vi "groups_and_names_query.vi"(8 "error in (no error)":errorcluster, 10 "Small?":bool, 11 "Constraints":T1 {"Estimate Quality" scale=0.0..5.0}) -> (0 "error out":errorcluster, 1 "Description":string, 2 "Groups":string[](array[string]), 3 "Names":string[](array[string]), 4 "Description Returned?":bool)   [LabVIEW 2015]
doc: "Returns all groups and experiments within the given constraints and (if there is only one group) returns a description of the group and all experiments within the constraints."
uses:
  User Interface/Controls/Constraints.ctl
  <userlib>/_OpenG.lib/array/array.llb/Remove Duplicates from 1D Array (String)__ogtk.vi
  <userlib>/_OpenG.lib/array/array.llb/Empty 2D Array (Variant)__ogtk.vi
  <vilib>/addons/database/_DB Variant To Data/Database Variant To Data.xnode
panel:
  out "Min-Max experiment settings query":string
  out "Names SQL Query":string
  out "Selected Group":string
  out "Groups SQL Query":string
  out "Description SQL Query":string
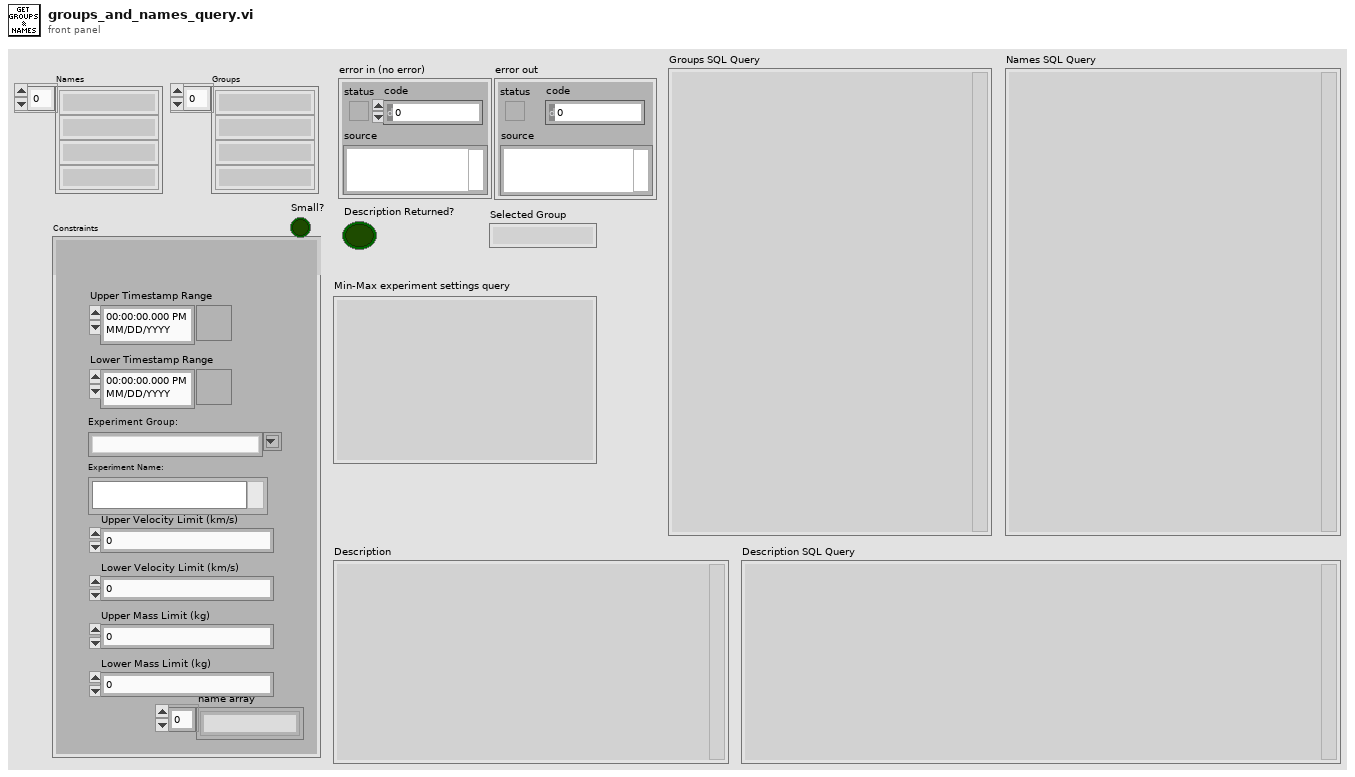
[diagram p1: front panel]
types:
  T1 = typedef "Constraints.ctl" = cluster{"Upper Timestamp Range":timestamp, "Lower Timestamp Range":timestamp, "Experiment Group:":string, "Experiment Name:":i32[], "Upper Velocity Limit (km/s)":dbl, "Lower Velocity Limit (km/s)":dbl, "Upper Mass Limit (kg)":dbl, "Lower Mass Limit (kg)":dbl, "name array":string[], "Estimate Quality":cluster{dbl, dbl}}
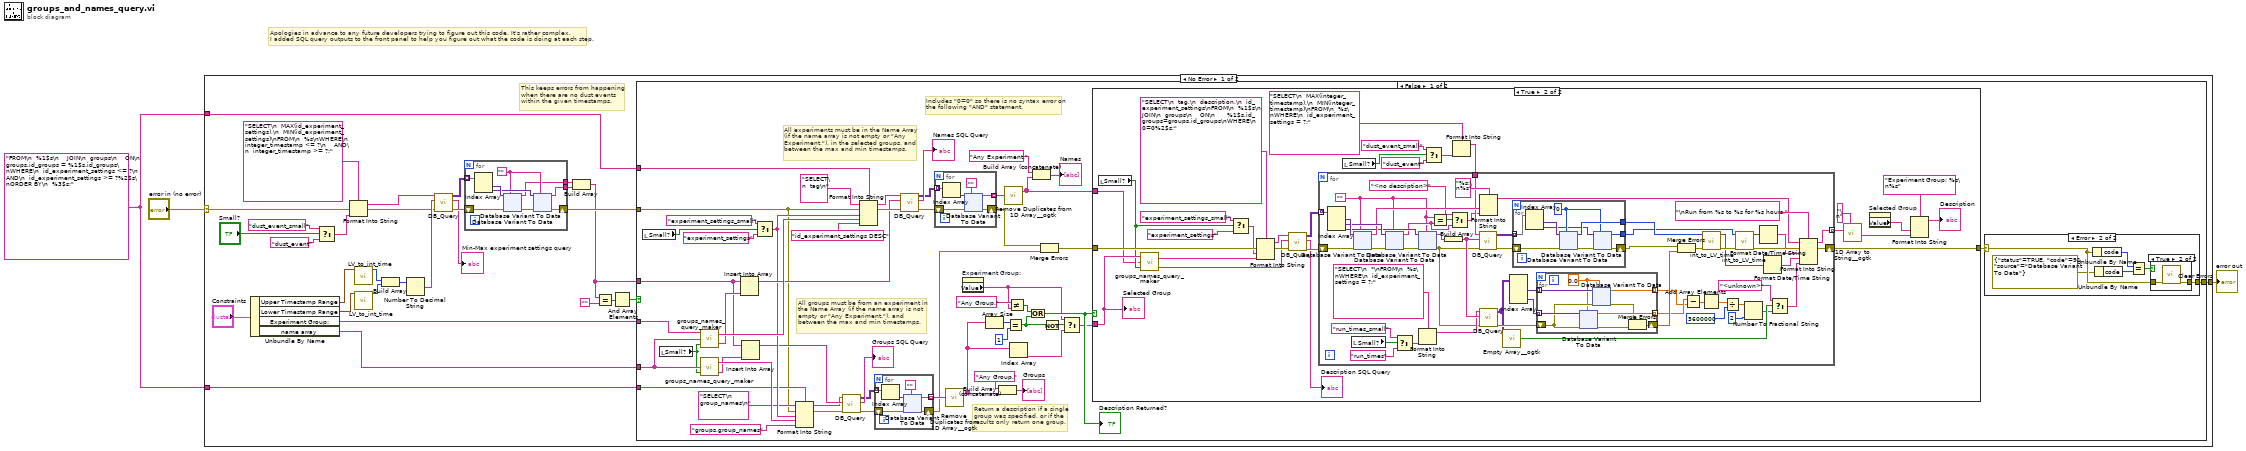
[diagram p0: block diagram]
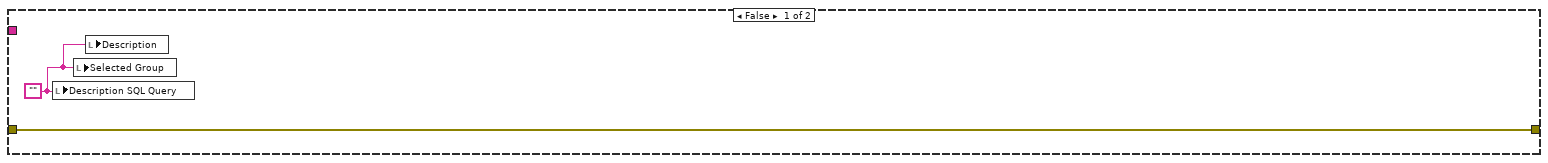
[diagram p4: hidden frame]
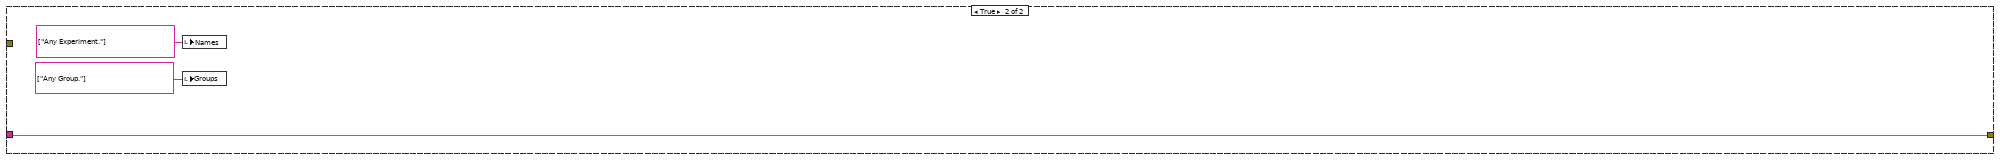
[diagram p5: hidden frame]
diagram:
  w1 = "FROM\n  %1$s\n    JOIN\n  groups\n    ON\n      groups.id_groups = %1$s.id_groups\nWHERE\n  id_experiment_settings <= ?\n    AND\n  id_experiment_settings >= ?%2$s\nORDER BY\n  %3$s;" ("format string")
  # "Apologies in advance to any future developers trying to figure out this code. It's rather complex.\nI added SQL query outputs to the front panel to help you figure out what the code is doing at each step."
  n1 = case shown="No Error" "error in (no error)" {
    selector: "error in (no error)" -> [w17 w578]
    tunnel: [w33 w578] -> w3
    tunnel: w1 -> [w22 _]
    tunnel: w1 -> [w21 _]
    frame No Error {
      # "This keeps errors from happening\nwhen there are no dust events\nwithin the given timestamps."
      n2 = Unbundle By Name("Constraints") -> ("Upper Timestamp Range"=w31:timestamp, "Lower Timestamp Range"=w32:timestamp, "Experiment Group:"=w20:string, "name array"=w29:string[])
      n3 = Select(t="dust_event_small", s="Small?", f="dust_event") -> (s? t:f=w18:string)
      n4 = Format Into String(format string="SELECT\n  MAX(id_experiment_settings),\n  MIN(id_experiment_settings)\nFROM\n  %s\nWHERE\n  integer_timestamp <= ?\n    AND\n  integer_timestamp >= ?;", error in=w17, w18) -> (resulting string=w15:string, error out=w14:errorcluster)  [unwired: 1 in]
      n5 = call "LV_to_int_time.vi"("Time Stamp"=w31) -> ("Integer Time"=w26:i64)  [unwired: 8 in, 1 out]
      n6 = call "LV_to_int_time.vi"("Time Stamp"=w32) -> ("Integer Time"=w25:i64)  [unwired: 8 in, 1 out]
      n7 = Build Array(w26, w25) -> (w24:i64[])
      n8 = Number To Decimal String(number=w24) -> (decimal integer string=w16:string[])  [unwired: 1 in]
      n9 = call "DB_Query.vi"("error in (no error)"=w14, "Parameters"=w16, "Parameterized Query"=w15) -> ("error out"=w13:errorcluster, "Query in Standard Format"=→"Min-Max experiment settings query":string, "Results"=w12:variant[][])  [unwired: 6 in]
      n10 = for {
        shift-right: [w507] -> w11
        shift-left: w13 -> [w512]
        tunnel: w12 -> [w513] mode=indexing
        tunnel: [w506] -> w10
        tunnel: [w505] -> w9
        w508 = "" ("t")
        n11 = Index Array(array=w513) -> (element #1=w511:variant, element #2=w509:variant)  [unwired: 2 in]
        n12 = xnode "Database Variant To Data"("database variant"=w511, "error in (no error)"=w512, "type"=w508) -> ("data"=w506:string, "error out"=w510:errorcluster)
        n13 = xnode "Database Variant To Data"("database variant"=w509, "error in (no error)"=w510, "type"=w508) -> ("data"=w505:string, "error out"=w507:errorcluster)
      }
      n14 = Build Array(w10, w9) -> (w7:string[])
      n15 = Equal?(x=w7, y="") -> (x = y?=w4:bool[])
      n16 = And Array Elements(Boolean array=w4) -> (logical AND=w5:bool)
      n17 = case shown="False" w5 {
        tunnel: [w87 w504] -> w33
        tunnel: w29 -> [w67 _]
        tunnel: w22 -> [w42 _]
        tunnel: w21 -> [w41 _]
        tunnel: w20 -> [w40 _]
        tunnel: w11 -> [w36 w504]
        tunnel: w7 -> [w35 _]
        frame False {
          # "Includes \"0=0\" so there is no syntax error on\nthe following \"AND\" statement."
          # "Return a description if a single\ngroup was specified, or if the\nresults only return one group."
          # "All groups must be from an experiment in\nthe Name Array (if the name array is not\nempty or \"Any Experiment.\"), and\nbetween the max and min timestamps."
          # "All experiments must be in the Name Array\n(if the name array is not empty or \"Any\nExperiment.\"), in the selected groups, and\nbetween the max and min timestamps."
          n18 = local read "Small?"() -> (w37:bool)
          n19 = local read "Small?"() -> (w38:bool)
          n20 = call "groups_names_query_maker.vi"("Small?"=w38, "Name Array"=w67) -> ("Parameters"=w54:string[], "Group and Names Query"=w55:string)  [unwired: 1 in]
          n21 = call "groups_names_query_maker.vi"("Small?"=w38, "Name Array"=w67, "Group  Name"=w40) -> ("Parameters"=w61:string[], "Group and Names Query"=w64:string)
          n22 = Insert Into Array(array=w35, new element=w61) -> (w58:string[])  [unwired: 1 in]
          n23 = Insert Into Array(array=w35, new element=w54) -> (w52:string[])  [unwired: 1 in]
          n24 = Select(t="experiment_settings_small", s=w37, f="experiment_settings") -> (s? t:f=w56:string)
          n25 = Format Into String(format string=w41, initial string="SELECT\n  group_names\n", error in=w36, w56, w55, "groups.group_names" ("input 4")) -> (resulting string=w51:string, error out=w53:errorcluster)
          n26 = call "DB_Query.vi"("error in (no error)"=w53, "Parameters"=w52, "Parameterized Query"=w51) -> ("error out"=w48:errorcluster, "Query in Standard Format"=→"Groups SQL Query":string, "Results"=w49:variant[][])  [unwired: 6 in]
          n27 = Format Into String(format string=w42, initial string="SELECT\n  tag\n", error in=w36, w56, w64, "id_experiment_settings DESC" ("input 4")) -> (resulting string=w63:string, error out=w62:errorcluster)
          n28 = for {
            tunnel: [w466] -> w84 mode=indexing
            shift-right: [w465] -> w81
            shift-left: w48 -> [w469]
            tunnel: w49 -> [w464] mode=indexing
            n29 = Index Array(array=w464) -> (element=w467:variant)  [unwired: 1 in]
            n30 = xnode "Database Variant To Data"("database variant"=w467, "error in (no error)"=w469, "type"="" ("t")) -> ("data"=w466:string, "error out"=w465:errorcluster)
          }
          n31 = call "DB_Query.vi"("error in (no error)"=w62, "Parameters"=w58, "Parameterized Query"=w63) -> ("error out"=w57:errorcluster, "Query in Standard Format"=→"Names SQL Query":string, "Results"=w59:variant[][])  [unwired: 6 in]
          n32 = for {
            tunnel: [w89] -> w85 mode=indexing
            shift-right: [w90] -> w82
            shift-left: w57 -> [w93]
            tunnel: w59 -> [w88] mode=indexing
            n33 = Index Array(array=w88) -> (element=w91:variant)  [unwired: 1 in]
            n34 = xnode "Database Variant To Data"("database variant"=w91, "error in (no error)"=w93, "type"="" ("t")) -> ("data"=w89:string, "error out"=w90:errorcluster)
          }
          n35 = call-poly <userlib>:"Remove Duplicates from 1D Array__ogtk.vi"("Input Array"=w84) -> ("Output Array"=w34:string[])  [unwired: 1 out]
          n36 = property on="Experiment Group:" class="CmbBox"() -> ("Value"=w39:string)  [unwired: 2 in, 2 out]
          n37 = Array Size(array=w34) -> (size(s)=w78:i32)
          n38 = Build Array (concatenate)("Any Group.", w34) -> (→"Groups":string[])
          n39 = call-poly <userlib>:"Remove Duplicates from 1D Array__ogtk.vi"("Input Array"=w85) -> ("Output Array"=w47:string[])  [unwired: 1 out]
          n40 = Equal?(x=w78, y=1) -> (x = y?=w71:bool)
          n41 = Not Equal?(x="Any Group.", y=w39) -> (x != y?=w74:bool)
          n42 = Index Array(array=w34) -> (element=w70:string)  [unwired: 1 in]
          n43 = Or(x=w74, y=w71) -> (x .or. y?=w72:bool)
          "Description Returned?" <- w72
          n44 = Build Array (concatenate)("Any Experiment.", w47) -> (→"Names":string[])
          n45 = Merge Errors(w82, w81) -> (w80:errorcluster)
          n46 = Not(x=w71) -> (.not. x?=w68:bool)
          n47 = Select(t=w39, s=w68, f=w70) -> (s? t:f=w69:string)
          n48 = case shown="True" w72 {
            tunnel: w80 -> [w137 w165]
            tunnel: [w137 w164] -> w79
            tunnel: w47 -> [_ w138]
            tunnel: w69 -> [_ w160]
            frame False {
              w136 = ""
              n49 = local write "Description SQL Query"(w136) -> ()
              n50 = local write "Selected Group"(w136) -> ()
              n51 = local write "Description"(w136) -> ()
            }
            frame True {
              n52 = local read "Small?"() -> (w156:bool)
              n53 = call "groups_names_query_maker.vi"("Small?"=w156, "Name Array"=w138, "Group  Name"=w160) -> ("Parameters"=w152:string[], "Group and Names Query"=w159:string)
              n54 = Select(t="experiment_settings_small", s=w156, f="experiment_settings") -> (s? t:f=w155:string)
              n55 = Format Into String(format string="SELECT\n  tag,\n  description,\n  id_experiment_settings\nFROM\n  %1$s\n    JOIN\n  groups\n    ON\n      %1$s.id_groups=groups.id_groups\nWHERE\n  0=0%2$s;" ("string"), error in=w165, w155, w159) -> (resulting string=w153:string, error out=w154:errorcluster)  [unwired: 1 in]
              n56 = call "DB_Query.vi"("error in (no error)"=w154, "Parameters"=w152, "Parameterized Query"=w153) -> ("error out"=w150:errorcluster, "Query in Standard Format"=→"Description SQL Query":string, "Results"=w151:variant[][])  [unwired: 6 in]
              n57 = local read "Small?"() -> (w144:bool)
              n58 = Select(t="dust_event_small", s=w144, f="dust_event") -> (s? t:f=w143:string)
              n59 = Format Into String(format string="SELECT\n  MAX(integer_timestamp),\n  MIN(integer_timestamp)\nFROM\n  %s\nWHERE\n  id_experiment_settings = ?;", w143) -> (resulting string=w139:string)  [unwired: 2 in, 1 out]
              n60 = for {
                shift-right: [w192] -> w164
                shift-left: w150 -> [w216]
                tunnel: w151 -> [w220] mode=indexing
                tunnel: [w190] -> w148 mode=indexing
                tunnel: w139 -> [w187]
                w168 = "" ("Integer Time")
                n61 = Index Array(array=w220) -> (element #1=w221:variant, element #2=w219:variant, element #3=w175:variant)  [unwired: 3 in]
                n62 = local read "Small?"() -> (w182:bool)
                n63 = xnode "Database Variant To Data"("database variant"=w221, "error in (no error)"=w216, "type"=w168) -> ("data"=w217:string, "error out"=w218:errorcluster)
                n64 = xnode "Database Variant To Data"("database variant"=w219, "error in (no error)"=w218, "type"=w168) -> ("data"=w170:string, "error out"=w176:errorcluster)
                n65 = Select(t="run_times_small", s=w182, f="run_times") -> (s? t:f=w179:string)
                n66 = xnode "Database Variant To Data"("database variant"=w175, "error in (no error)"=w176, "type"=w168) -> ("data"=w173:string, "error out"=w174:errorcluster)
                n67 = Format Into String(format string="SELECT\n  *\nFROM\n  %s\nWHERE\n  id_experiment_settings = ?;", w179) -> (resulting string=w177:string)  [unwired: 2 in, 1 out]
                n68 = Equal?(x=w168, y=w170) -> (x = y?=w171:bool)
                n69 = Build Array(w173) -> (w186:string[])
                n70 = Select(t="<no description>", s=w171, f=w170) -> (s? t:f=w172:string)
                n71 = call "DB_Query.vi"("error in (no error)"=w174, "Parameters"=w186, "Parameterized Query"=w187) -> ("error out"=w185:errorcluster, "Results"=w183:variant[][])  [unwired: 6 in, 1 out]
                n72 = Format Into String(format string="%s:\n%s", w217, w172) -> (resulting string=w194:string)  [unwired: 2 in, 1 out]
                n73 = call "DB_Query.vi"("error in (no error)"=w174, "Parameters"=w186, "Parameterized Query"=w177) -> ("error out"=w189:errorcluster, "Results"=w188:variant[][])  [unwired: 6 in, 1 out]
                n74 = call-poly <userlib>:"Empty Array__ogtk.vi"("Array"=w188) -> ("Empty Array?"=w209:bool)  [unwired: 8 in]
                n75 = Index Array(array=w188) -> (element #1=w215:variant[], element #2=w214:variant[])  [unwired: 4 in]
                n76 = for {
                  tunnel: [w261] -> w195
                  shift-right: [w258] -> w202
                  shift-left: w185 -> [w260]
                  tunnel: [w255] -> w184
                  tunnel: w183 -> [w254] mode=indexing
                  w257 = i64 0
                  n77 = Index Array(array=w254) -> (element #1=w262:variant, element #2=w256:variant)  [unwired: 2 in]
                  n78 = xnode "Database Variant To Data"("database variant"=w262, "error in (no error)"=w260, "type"=w257) -> ("data"=w261:i64, "error out"=w259:errorcluster)
                  n79 = xnode "Database Variant To Data"("database variant"=w256, "error in (no error)"=w259, "type"=w257) -> ("data"=w255:i64, "error out"=w258:errorcluster)
                }
                n80 = for {
                  tunnel: w215 -> [w335] mode=indexing
                  tunnel: w214 -> [w334] mode=indexing
                  tunnel: [w331] -> w205 mode=indexing
                  tunnel: [w333] -> w204 mode=indexing
                  shift-right: [w328] -> w206
                  shift-left: w189 -> [w332]
                  w327 = 0.0
                  n81 = xnode "Database Variant To Data"("database variant"=w334, "error in (no error)"=w332, "type"=w327) -> ("data"=w331:dbl, "error out"=w329:errorcluster)
                  n82 = xnode "Database Variant To Data"("database variant"=w335, "error in (no error)"=w332, "type"=w327) -> ("data"=w333:dbl, "error out"=w330:errorcluster)
                  n83 = Merge Errors(w330, w329) -> (w328:errorcluster)
                }
                n84 = Merge Errors(w202, w206) -> (w193:errorcluster)
                n85 = Subtract(x=w205, y=w204) -> (x-y=w203:dbl[])
                n86 = Add Array Elements(numeric array=w203) -> (sum=w213:dbl)
                n87 = call "int_to_LV_time.vi"("error in (no error)"=w193, "Integer Timestamp"=w195) -> ("error out"=w197:errorcluster, "time stamp"=w167:timestamp)  [unwired: 7 in]
                n88 = Divide(x=w213, y=i64 3600000) -> (x/y=w211:dbl)
                n89 = call "int_to_LV_time.vi"("error in (no error)"=w197, "Integer Timestamp"=w184) -> ("error out"=w201:errorcluster, "time stamp"=w166:timestamp)  [unwired: 7 in]
                n90 = Number To Fractional String(number=w211, precision (6)=i16 2) -> (F-format string=w208:string)  [unwired: 2 in]
                n91 = Format Date/Time String(seconds (now)=w166) -> (date/time string=w199:string)  [unwired: 2 in]
                n92 = Format Date/Time String(seconds (now)=w167) -> (date/time string=w200:string)  [unwired: 2 in]
                n93 = Select(t="<unknown>" ("f"), s=w209, f=w208) -> (s? t:f=w196:string)
                n94 = Format Into String(format string="\nRun from %s to %s for %s hours.", initial string=w194, error in=w201, w199, w200, w196) -> (resulting string=w190:string, error out=w192:errorcluster)
              }
              n95 = call <userlib>:"1D Array to String__ogtk.vi"("delimiter (Tab)"="\n", "Array of Strings"=w148) -> ("delimited string"=w147:string)  [unwired: 9 in]
              n96 = property on="Selected Group" class="Str"() -> ("Value"=w162:string)  [unwired: 2 in, 2 out]
              n97 = Format Into String(format string="Experiment Group: %s\n%s", w162, w147) -> (resulting string=→"Description":string)  [unwired: 2 in, 1 out]
              "Selected Group" <- w160
            }
          }
          n98 = case shown="Error" w79 {
            selector: w79 -> [w126 w131]
            tunnel: [w126 w132] -> w87
            frame No Error {
            }
            frame Error {
              n99 = Unbundle By Name(w131) -> ("code"=w129:i32)
              n100 = Unbundle By Name(errorcluster {"status"=TRUE, "code"=91, "source"="Database Variant To Data"} ("error out")) -> ("code"=w128:i32)
              n101 = Equal?(x=w129, y=w128) -> (x = y?=w127:bool)
              n102 = case shown="True" w127 {
                tunnel: [w133 w134] -> w132
                tunnel: w131 -> [w133 w135]
                frame False {
                }
                frame True {
                  n103 = call <vilib>:"Clear Errors.vi"("error in (no error)"=w135) -> ("error out"=w134:errorcluster)  [unwired: 5 in, 1 out]
                }
              }
            }
          }
        }
        frame True {
          n104 = local write "Groups"(string[] ["Any Group."] ("Names")) -> ()
          n105 = local write "Names"(string[] ["Any Experiment."] ("Names")) -> ()
        }
      }
    }
    frame Error {
    }
  }
  "error out" <- w3
